vi "Dice throwing.vi"() -> ()   [LabVIEW 2020]
panel:
  out "Dice":u16(ring)
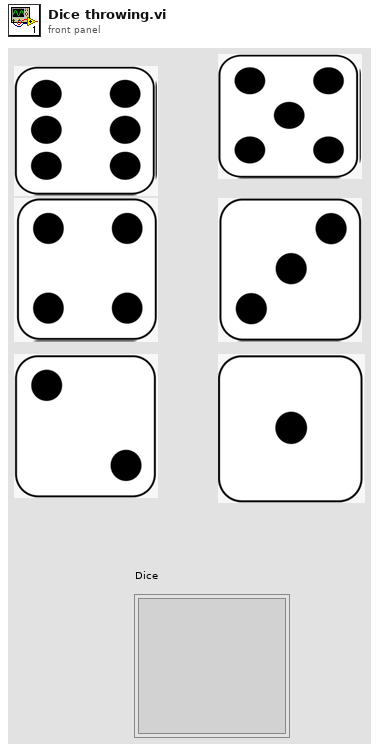
[diagram p1: front panel]
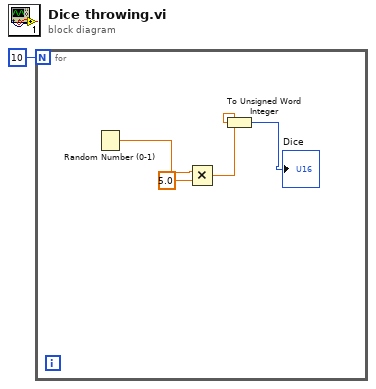
[diagram p0: block diagram]
diagram:
  n1 = for {
    N: 10 -> [_]
    n2 = Random Number (0-1)() -> (number: 0 to 1=w5:dbl)
    n3 = Multiply(x=w5, y=5.0) -> (x*y=w3:dbl)
    n4 = To Unsigned Word Integer(number=w3) -> (unsigned 16bit integer=→"Dice":u16)
  }
